vi "Close.vi"(8 "error":errorcluster, 11 "VISA name":refnum<visa-resource-name>) -> (0 "error out":errorcluster)   [LabVIEW 2025, in "TDK-Lambda GEN LAN Series.lvlib"]
doc: "Closes the I/O interface with the Genesys Power Supply."
uses:
  <userlib>/TDK-Lambda GEN LAN Series/TDK-Lambda GEN LAN Series.lvlib
panel:
  # "TDK-Lambda Genesys \n LAN\n  DC Power Supplies"
  # "Close Instrument Port"
  # "(c) 2019 TDK-Lambda.  ALL RIGHTS RESERVED."
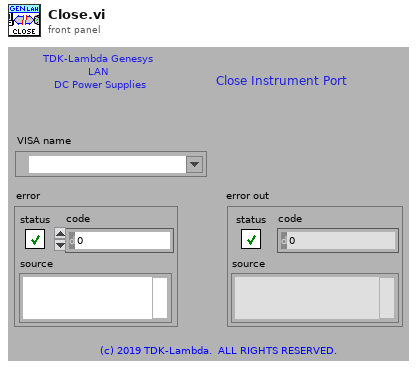
[diagram p1: front panel]
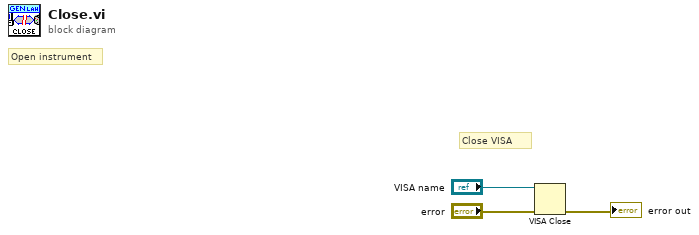
[diagram p0: block diagram]
diagram:
  # "Close VISA"
  # "Open instrument"
  n1 = VISA Close(VISA resource name="VISA name", error in (no error)="error") -> (error out=→"error out":errorcluster)
